vi "Tempo do servidor.vi"(8 "error in (no error)":errorcluster, 11 "Connection in":T1) -> (0 "error out":errorcluster, 1 "time stamp":timestamp, 3 "Connection out":T1)   [LabVIEW 2020, in "PostgreSQL Driver.lvlib"]
uses:
  PostgreSQL Driver.lvlib
  <vilib>/addons/database/Connection.llb/Conn ObjectReference.ctl
  <vilib>/addons/database/NI_Database_API.lvlib
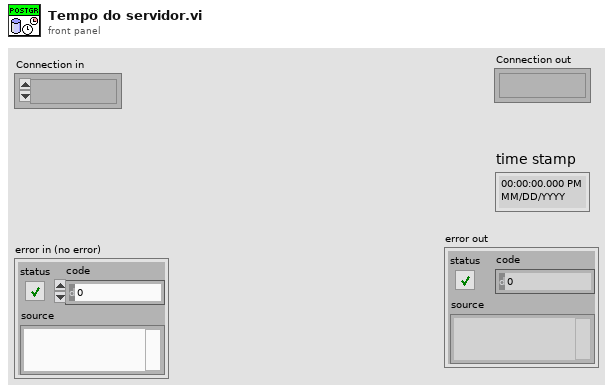
[diagram p1: front panel]
types:
  T1 = typedef "NI_Database_API.lvlib/Conn ObjectReference.ctl" = refnum<k1>
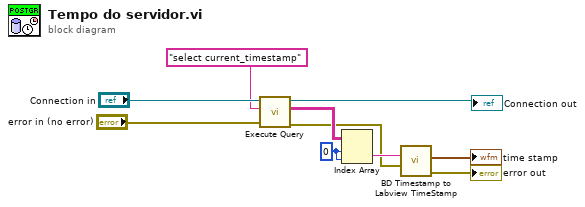
[diagram p0: block diagram]
diagram:
  w6 = 0 ("index (row)")
  n1 = call "Execute Query.vi"("error in (no error)"="error in (no error)", "SQL query"="select current_timestamp", "Connection in"="Connection in") -> ("error out"=w2:errorcluster, "data"=w7:string[][], "Connection out"=→"Connection out":T1)  [unwired: 3 in, 3 out]
  n2 = Index Array(array=w7, index (row)=w6, index (col)=w6) -> (element=w4:string)
  n3 = call "BD Timestamp to Labview TimeStamp.vi"("error in"=w2, "BD Time Stamp"=w4) -> ("error out"=→"error out":errorcluster, "time stamp"=→"time stamp":timestamp)  [unwired: 4 in]
